vi "串口数据.vi"(1 "串口输入":T1, 9 "报文最大值":u16=1200, 12 "枚举":T2(ring)) -> (15 "串口记录":T1)   [LabVIEW 2019, in "MainPage.lvlib" / "MainPage.lvclass"]
uses:
  MainPage.lvclass
panel:
  # "由于闪退问题弃用值引用\n改用功能全局"
  # "感觉可能会存在故障"
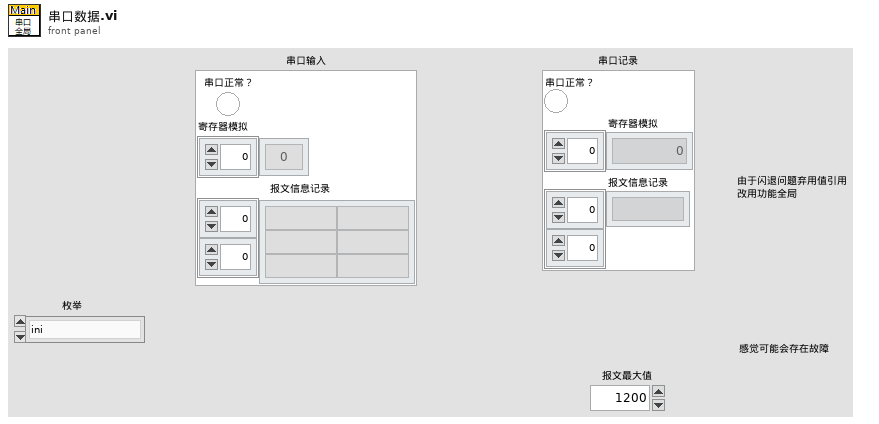
[diagram p1: front panel]
types:
  T1 = cluster{"串口正常？":bool, "寄存器模拟":u16[], "报文信息记录":string[][]}
  T2 = enum16{"ini", "读取", "写入-报文记录", "写入-寄存器模拟", "写入-串口状态", "增加报文记录"}
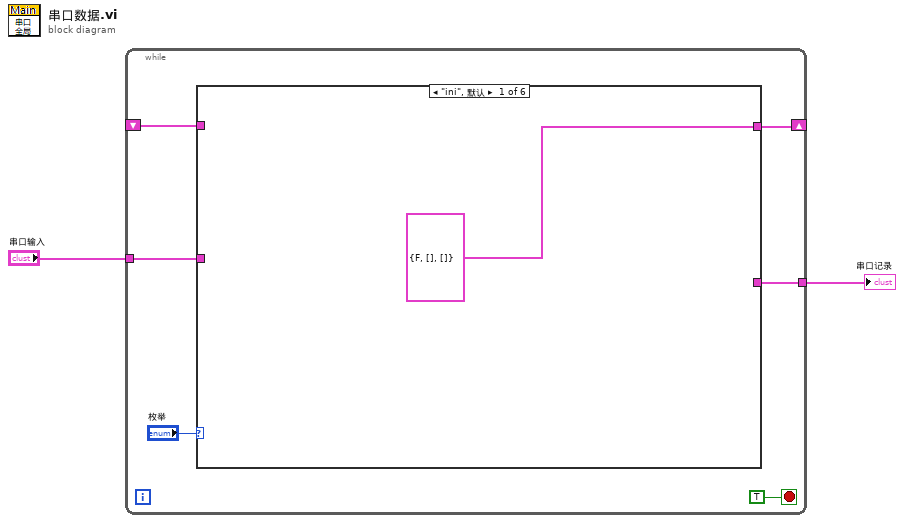
[diagram p0: block diagram]
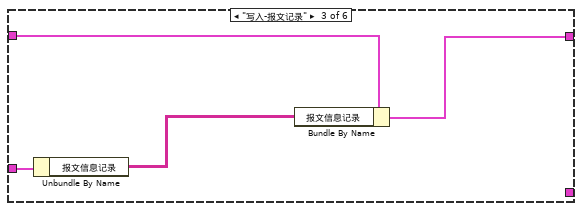
[diagram p3: hidden frame]
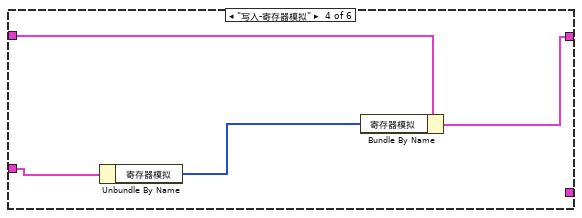
[diagram p4: hidden frame]
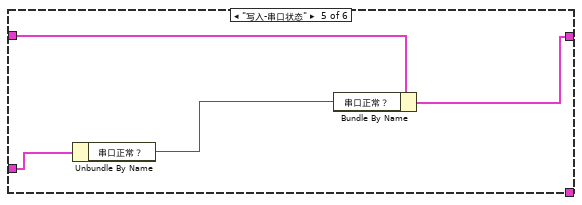
[diagram p5: hidden frame]
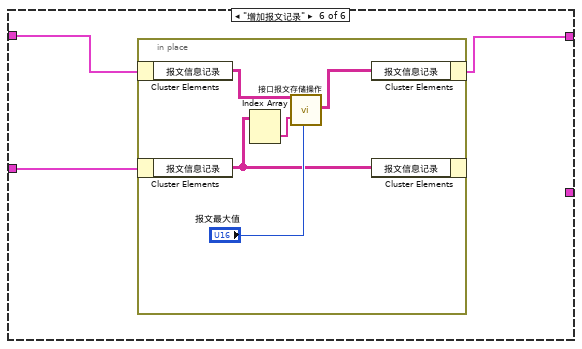
[diagram p6: hidden frame]
diagram:
  n1 = while {
    shift-right: [w6] -> _
    shift-left: _ -> [w5]
    tunnel: "串口输入" -> [w4]
    tunnel: [w3] -> w1
    stop <- TRUE stop-if-true
    n2 = case shown="\"ini\", 默认" "枚举" {
      tunnel: [T1 {"串口正常？"=FALSE, "寄存器模拟"=[], "报文信息记录"=[]} ("串口反馈") w10 w13 w15 w21 w23] -> w6
      tunnel: w5 -> [_ w10 w14 w16 w20 w24]
      tunnel: w4 -> [_ _ w12 w17 w19 w25]
      tunnel: [_ w10 _ _ _ _] -> w3
      frame "ini", Default {
      }
      frame "读取" {
      }
      frame "写入-报文记录" {
        n3 = Unbundle By Name(w12) -> ("报文信息记录"=w11:string[][])
        n4 = Bundle By Name(cluster=w14, "报文信息记录"=w11) -> (w13:T1)
      }
      frame "写入-寄存器模拟" {
        n5 = Unbundle By Name(w17) -> ("寄存器模拟"=w18:u16[])
        n6 = Bundle By Name(cluster=w16, "寄存器模拟"=w18) -> (w15:T1)
      }
      frame "写入-串口状态" {
        n7 = Unbundle By Name(w19) -> ("串口正常？"=w22:bool)
        n8 = Bundle By Name(cluster=w20, "串口正常？"=w22) -> (w21:T1)
      }
      frame "增加报文记录" {
        n9 = in-place {
          n10 = in-place-cluster #1(w24) -> ("报文信息记录"=w30:string[][])
          n11 = in-place-cluster #2(w25) -> ("报文信息记录"=w27:string[][])
          n12 = Index Array(array=w27) -> (element=w26:string[])  [unwired: 2 in]
          n13 = call "接口报文存储操作.vi"("原始记录"=w30, "报文信息"=w26, "报文最大量"="报文最大值") -> ("输出记录"=w29:string[][])  [unwired: 16 in]
          n14 = in-place-cluster #1("报文信息记录"=w29) -> (w23:T1)
          n15 = in-place-cluster #2("报文信息记录"=w27) -> ()  [unwired: 1 out]
        }
      }
    }
  }
  "串口记录" <- w1
